vi "Set Macro by Index.vi"(8 "error in (no error)":errorcluster, 9 "TriggerAction Q.lvclass":refnum<class "TriggerAction Q.lvclass">, 10 "Index":i32, 11 "Motions in":refnum<class "Motions.lvclass">) -> (0 "error out":errorcluster, 2 "replaced":bool, 3 "Motions out":refnum<class "Motions.lvclass">)   [LabVIEW 2016, in "Hardware.lvlib" / "Motions.lvlib" / "Motions.lvclass"]
uses:
  <userlib>/Common Components/Hardware/Abstract System/Motions/Motions/Motions.lvclass
  <userlib>/Common Components/TriggerAction Q/TriggerAction Q/TriggerAction Q.lvclass
  <userlib>/Common Components/Hardware/Abstract System/Motions/Motions/Motions.lvclass/Motions.ctl
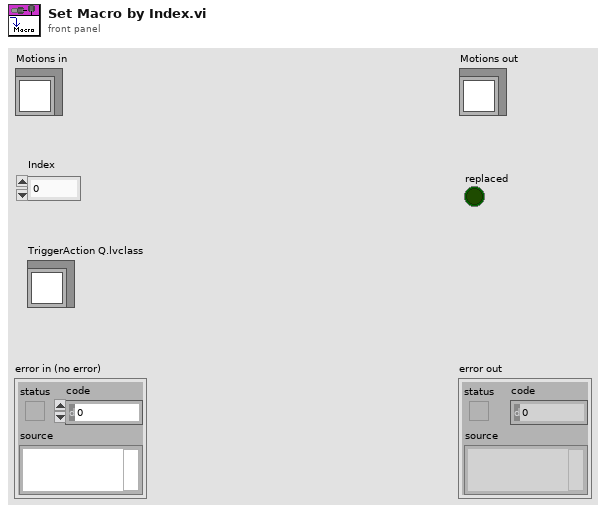
[diagram p1: front panel]
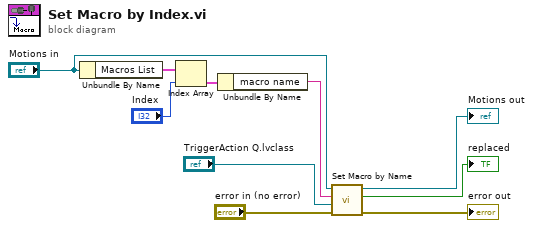
[diagram p0: block diagram]
diagram:
  n1 = Unbundle By Name("Motions in") -> ("Macros List"=w10:cluster{"enabled?":bool, "macro name":string}[])
  n2 = Index Array(array=w10, index="Index") -> (element=w8:cluster{"enabled?":bool, "macro name":string})
  n3 = Unbundle By Name(w8) -> ("macro name"=w5:string)
  n4 = call <userlib>:"Set Macro by Name.vi"("error in (no error)"="error in (no error)", "TriggerAction Q.lvclass"="TriggerAction Q.lvclass", "Macro Name"=w5, "Motions in"="Motions in") -> ("error out"=→"error out":errorcluster, "replaced"=→"replaced":bool, "Motions out"=→"Motions out":refnum<class "Motions.lvclass">)  [unwired: 5 in]
